vi "PenaltyPosSkillVSS.vi"(8 "error in (no error)":errorcluster, 9 "Game":refnum<class "Game.lvclass">, 10 "Robot in":refnum<class "Robot.lvclass">, 11 "PenaltyPosSkillVSS in":refnum<class "PenaltyPosSkillVSS.lvclass">) -> (0 "error out":errorcluster, 2 "Robot out":refnum<class "Robot.lvclass">, 3 "PenaltyPosSkillVSS out":refnum<class "PenaltyPosSkillVSS.lvclass">)   [LabVIEW 2023, in "PenaltyPosSkillVSS.lvclass"]
uses:
  PenaltyPosSkillVSS.lvclass
  Robot_class/Robot.lvclass
  Game_class/Game.lvclass
  Game_class/Game.lvclass/Game.ctl
  Robot_class/Robot.lvclass/Robot.ctl
  Game_class/Read FieldRef.vi
  Robot_class/Write dest_x.vi
  Robot_class/Write dest_y.vi
  Field_class/Field.lvclass
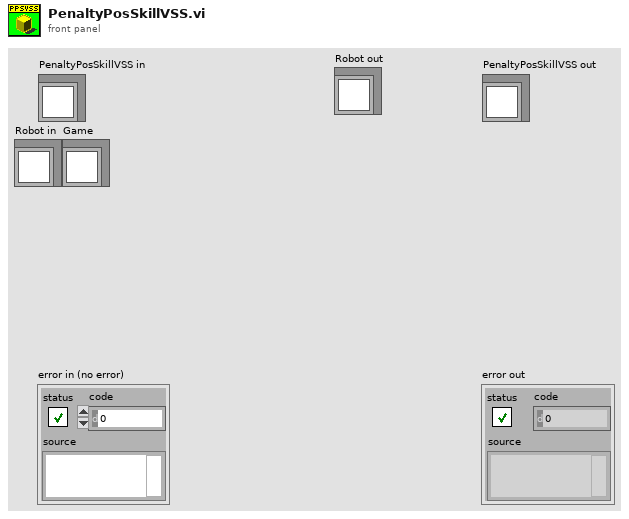
[diagram p1: front panel]
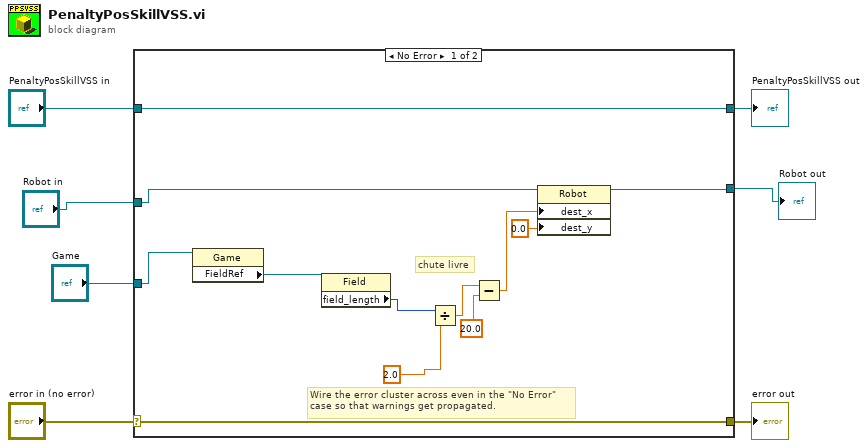
[diagram p0: block diagram]
diagram:
  n1 = case shown="No Error" "error in (no error)" {
    selector: "error in (no error)" -> [w18 w22]
    tunnel: [w18 w22] -> w6
    tunnel: [w19 w21] -> w4
    tunnel: "PenaltyPosSkillVSS in" -> [w19 w21]
    tunnel: "Robot in" -> [w17 w20]
    tunnel: "Game" -> [w15 _]
    tunnel: [w16 w20] -> w1
    frame No Error {
      # "chute livre"
      # "Wire the error cluster across even in the \"No Error\"\ncase so that warnings get propagated."
      n2 = property class="Game"(reference=w15) -> ("FieldRef"=w14:refnum<class "Field.lvclass">)  [unwired: 1 in, 2 out]
      n3 = property class="Field"(reference=w14) -> ("field_length"=w12:i32)  [unwired: 1 in, 2 out]
      n4 = Divide(x=w12, y=2.0) -> (x/y=w9:dbl)
      n5 = Subtract(x=w9, y=20.0 ("x")) -> (x-y=w10:dbl)
      n6 = property class="Robot"(reference=w17, "dest_x"=w10, "dest_y"=0.0 ("y")) -> (reference out=w16:refnum<class "Robot.lvclass">)  [unwired: 1 in, 1 out]
    }
    frame Error {
    }
  }
  "error out" <- w6
  "PenaltyPosSkillVSS out" <- w4
  "Robot out" <- w1
